vi "createSafeSheetName.vi"(7 "MS-Excel in":refnum<class "MS-Excel.lvclass">, 8 "error in (no error)":errorcluster, 11 "nameProposal":string) -> (0 "error out":errorcluster, 3 "SafeSheetName":string)   [LabVIEW 2017, in "LabVIEW NPOI.lvlib" / "MS-Excel.lvclass"]
doc: "Helper method to create a valid sheet name, which is conform to the rules, based on <b>nameProposal</b>. If <b>nameProposal</b> is empty this VI returns \"empty\" as <b>SafeSheetName</b>.\nRules:\n - never null\n - minimum length is 1\n - maximum length is 31\n - doesn't contain special chars: : 0x0000, 0x0003, / \\ ? * ] [\n - Sheet names must not begin or end with ' (apostrophe)\nInvalid characters are replaced by one space character ' '."
uses:
  MS-Excel.lvclass
  C:/Users/Neo/Desktop/Dev_Tools_BR/LabVIEW_NPOI/src/lib/NPOI 2.1.1/NPOI.dll
  lib/NPOI 2.1.1/NPOI.dll
  Get Sheet Count.vi
  Get Sheet List.vi
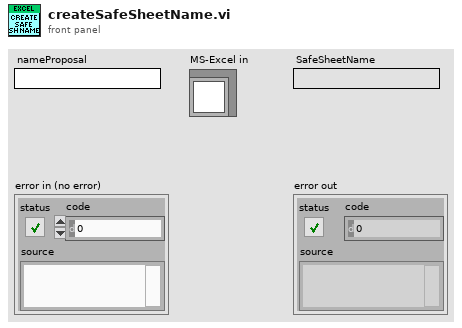
[diagram p1: front panel]
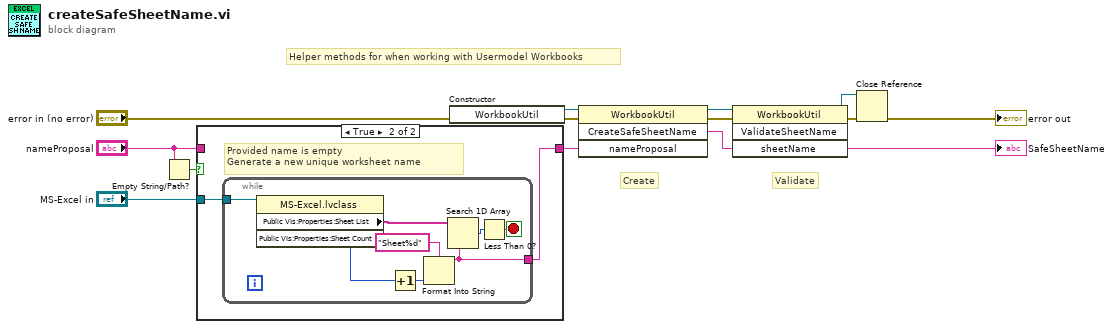
[diagram p0: block diagram]
diagram:
  # "Validate"
  # "Create"
  # "Helper methods for when working with Usermodel Workbooks"
  n1 = Empty String/Path?(string/path="nameProposal") -> (empty?=w3:bool)
  n2 = case shown="True" w3 {
    tunnel: "MS-Excel in" -> [_ w16]
    tunnel: "nameProposal" -> [w14 _]
    tunnel: [w14 w15] -> w1
    frame False {
    }
    frame True {
      # "Provided name is empty\nGenerate a new unique worksheet name"
      n3 = while {
        tunnel: w16 -> [w24]
        tunnel: [w17] -> w15
        stop <- w19 stop-if-true
        n4 = property class="MS-Excel.lvclass"(reference=w24) -> ("Public VIs:Properties:Sheet List"=w18:string[], "Public VIs:Properties:Sheet Count"=w23:i32)  [unwired: 1 in, 2 out]
        n5 = Increment(x=w23) -> (x+1=w22:i32)
        n6 = Format Into String(format string="Sheet%d", w22) -> (resulting string=w17:string)  [unwired: 2 in, 1 out]
        n7 = Search 1D Array(1D array=w18, element=w17) -> (index of element=w20:i32)  [unwired: 1 in]
        n8 = Less Than 0?(x=w20) -> (x < 0?=w19:bool)
      }
    }
  }
  n9 = constructor class="WorkbookUtil"(error in="error in (no error)") -> (reference out=w5:refnum<k24>, error out=w10:errorcluster)  [unwired: 2 in, 1 out]
  n10 = invoke class="WorkbookUtil" method="CreateSafeSheetName"(reference=w5, error in=w10, "nameProposal"=w1) -> (reference out=w9:refnum<k24>, error out=w7:errorcluster, "CreateSafeSheetName"=w11:string)  [unwired: 1 in, 1 out]
  "SafeSheetName" <- w11
  n11 = invoke class="WorkbookUtil" method="ValidateSheetName"(reference=w9, error in=w7, "sheetName"=w11) -> (reference out=w8:refnum<k24>, error out=w6:errorcluster)  [unwired: 1 in, 2 out]
  n12 = Close Reference(reference=w8, error in (no error)=w6) -> (error out=→"error out":errorcluster)
